vi "Get requst ID or error.vi"(8 "error in (no error)":errorcluster, 11 "IHandleUnsubscribed MsgPack in":refnum<class "IHandleUnsubscribed MsgPack.lvclass">) -> (0 "error out":errorcluster, 1 "ErrorOrSuccess":refnum<class "ErrorOrSuccess.lvclass">, 2 "Unsubscription Request ID":u64, 3 "IHandleUnsubscribed MsgPack out":refnum<class "IHandleUnsubscribed MsgPack.lvclass">)   [LabVIEW 2020, in "wamplv.lvlib" / "IHandleUnsubscribed MsgPack.lvclass"]
uses:
  IHandleUnsubscribed MsgPack.lvclass
  IHandleUnsubscribed MsgPack.lvclass/IHandleUnsubscribed MsgPack.ctl
  Message loop classes/ErrorOrSuccess/ErrorOrSuccess.lvclass
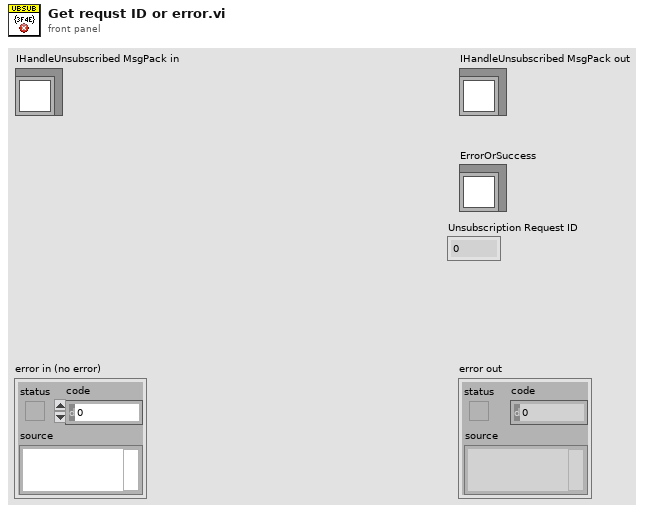
[diagram p1: front panel]
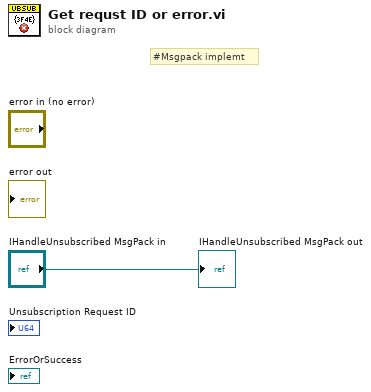
[diagram p0: block diagram]
diagram:
  # "#Msgpack implemt"
  "IHandleUnsubscribed MsgPack out" <- "IHandleUnsubscribed MsgPack in"
